vi "cdex - update quadcopter 3D model.vi"(5 "Y":sgl(slide) scale=-5.0..5.0, 7 "X":sgl(slide) scale=-5.0..5.0, 8 "Height":dbl(slide)=1.0 scale=0.0..4.0, 9 "Yaw":dbl(knob) scale=-6.28..6.28, 10 "Roll":dbl(knob) scale=-6.28..6.28, 11 "Pitch":dbl(knob) scale=-6.28..6.28) -> (3 "3D Picture Control":refnum<vi>(3d-picture))   [LabVIEW 2015]
uses:
  <vilib>/Analysis/1siggen.llb/Ramp Pattern by Samples.vi
  <vilib>/picture/3D Picture Control/NI_3D Picture Control.lvlib
  <vilib>/Analysis/NI_AALBase.lvlib
panel:
  # "Deploying Real-Time Math with NI LabVIEW"
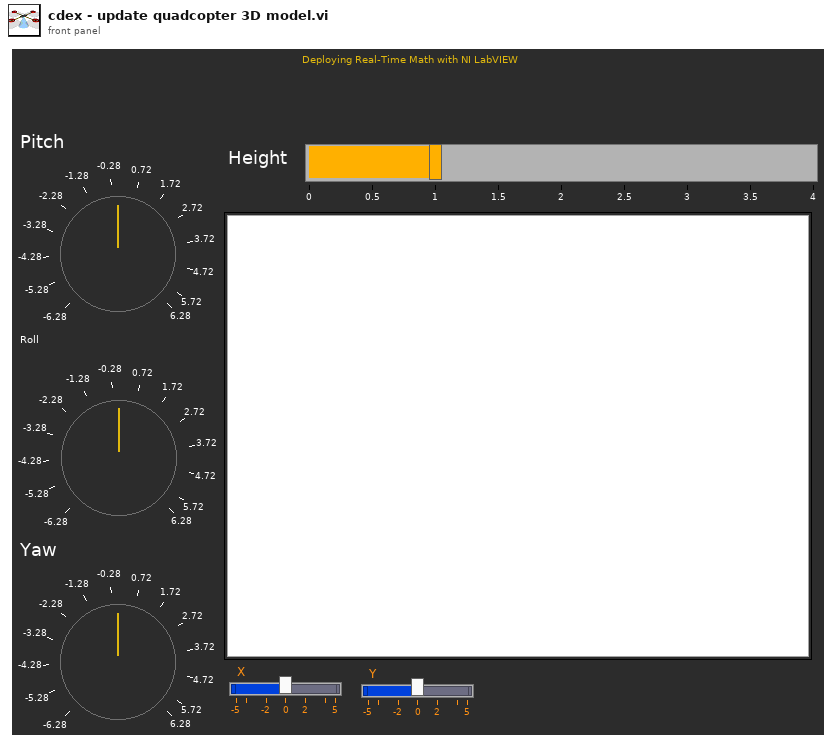
[diagram p1: front panel]
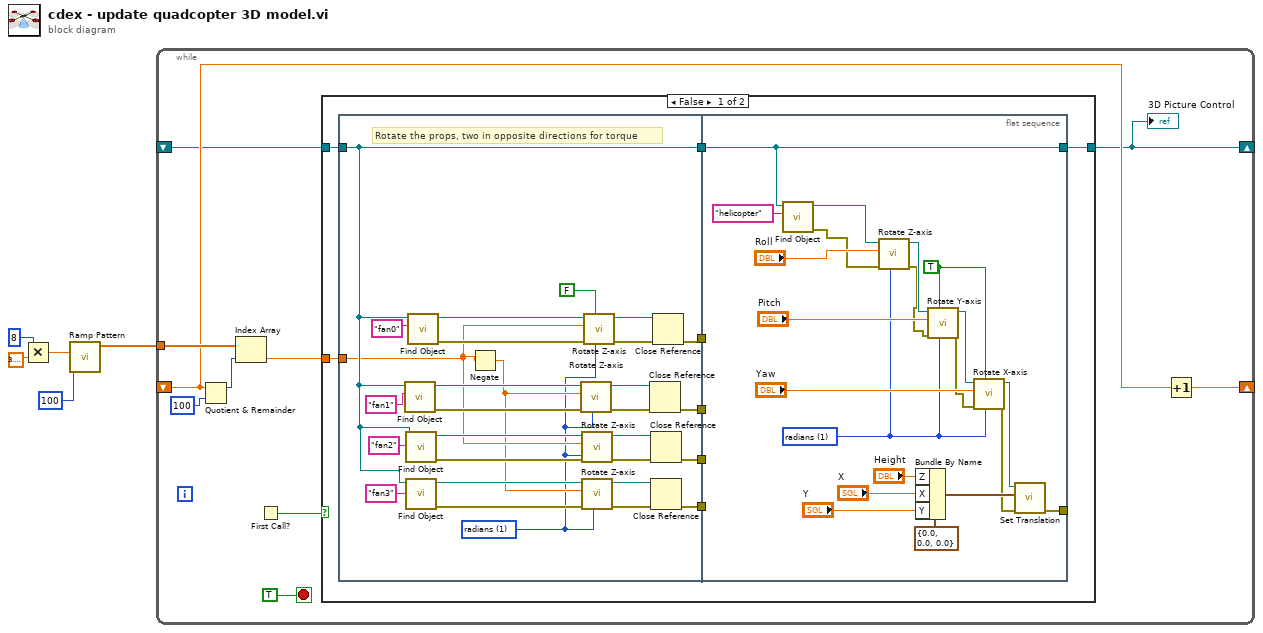
[diagram p0: block diagram]
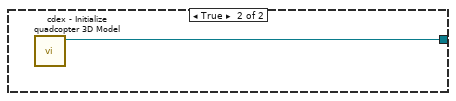
[diagram p2: hidden frame]
diagram:
  n1 = Multiply(x=8, y=3.141592653589793) -> (x*y=w3:dbl)
  n2 = call-poly <vilib>:"Ramp Pattern.vi"("end"=w3, "samples"=100) -> ("Ramp Pattern"=w1:dbl[])  [unwired: 8 in, 1 out]
  n3 = while {
    tunnel: w1 -> [w14]
    shift-right: [w11] -> _
    shift-left: _ -> [w10]
    shift-right: [w6] -> _
    shift-left: _ -> [w9]
    stop <- TRUE stop-if-true
    n4 = Quotient & Remainder(x=w10, y=100) -> (x-y*floor(x/y)=w13:i32)  [unwired: 1 out]
    n5 = Index Array(array=w14, index=w13) -> (element=w12:dbl)
    n6 = First Call?() -> (First Call?: T/F=w7:bool)
    n7 = case shown="False" w7 {
      tunnel: w9 -> [w22 _]
      tunnel: w12 -> [w21 _]
      tunnel: [w20 w74] -> w6
      frame False {
        n8 = flat-sequence {
          tunnel: w22 -> [w31]
          tunnel: [w31] -> w23
          tunnel: w21 -> [w30]
          tunnel: [w27] -> w19
          tunnel: [w26] -> w18
          tunnel: [w25] -> w17
          tunnel: [w24] -> w16
          tunnel: [w58] -> w20
          tunnel: w23 -> [w58]
          tunnel: w19 -> [_]
          tunnel: w18 -> [_]
          tunnel: w17 -> [_]
          tunnel: w16 -> [_]
          tunnel: [w53] -> _
          frame #0 {
            w28 = u16 1 items=["degree", "radians"] ("angle unit")
            # "Rotate the props, two in opposite directions for torque"
            n9 = call <vilib>:"Find Object.vi"("Object Name"="fan1", "Scene Refnum"=w31) -> ("error out"=w44:errorcluster, "Object Refnum"=w43:refnum<vi>)  [unwired: 8 in]
            n10 = call <vilib>:"Find Object.vi"("Object Name"="fan2", "Scene Refnum"=w31) -> ("error out"=w41:errorcluster, "Object Refnum"=w42:refnum<vi>)  [unwired: 8 in]
            n11 = call <vilib>:"Find Object.vi"("Object Name"="fan3", "Scene Refnum"=w31) -> ("error out"=w36:errorcluster, "Object Refnum"=w35:refnum<vi>)  [unwired: 8 in]
            n12 = call <vilib>:"Find Object.vi"("Object Name"="fan0", "Scene Refnum"=w31) -> ("error out"=w50:errorcluster, "Object Refnum"=w52:refnum<vi>)  [unwired: 8 in]
            n13 = Negate(x=w30) -> (-x=w29:dbl)
            n14 = call <vilib>:"Rotate Z-axis.vi"("angle unit"=w28, "error in (no error)"=w44, "angle"=w29, "Scene Object In"=w43) -> ("error out"=w46:errorcluster, "Scene Object Out"=w45:refnum<vi>)  [unwired: 6 in]
            n15 = call <vilib>:"Rotate Z-axis.vi"("angle unit"=w28, "error in (no error)"=w41, "angle"=w30, "Scene Object In"=w42) -> ("error out"=w39:errorcluster, "Scene Object Out"=w40:refnum<vi>)  [unwired: 6 in]
            n16 = call <vilib>:"Rotate Z-axis.vi"("angle unit"=w28, "error in (no error)"=w36, "angle"=w29, "Scene Object In"=w35) -> ("error out"=w38:errorcluster, "Scene Object Out"=w37:refnum<vi>)  [unwired: 6 in]
            n17 = call <vilib>:"Rotate Z-axis.vi"("angle unit"=w28, "Relative?"=FALSE, "error in (no error)"=w50, "angle"=w30, "Scene Object In"=w52) -> ("error out"=w47:errorcluster, "Scene Object Out"=w49:refnum<vi>)  [unwired: 5 in]
            n18 = Close Reference(reference=w45, error in (no error)=w46) -> (error out=w25:errorcluster)
            n19 = Close Reference(reference=w40, error in (no error)=w39) -> (error out=w26:errorcluster)
            n20 = Close Reference(reference=w37, error in (no error)=w38) -> (error out=w27:errorcluster)
            n21 = Close Reference(reference=w49, error in (no error)=w47) -> (error out=w24:errorcluster)
          }
          frame #1 {
            w59 = TRUE ("Relative?")
            w60 = u16 1 items=["degree", "radians"] ("angle unit")
            n22 = call <vilib>:"Find Object.vi"("Object Name"="helicopter", "Scene Refnum"=w58) -> ("error out"=w57:errorcluster, "Object Refnum"=w61:refnum<vi>)  [unwired: 8 in]
            n23 = call <vilib>:"Rotate Z-axis.vi"("angle unit"=w60, "error in (no error)"=w57, "angle"="Roll", "Scene Object In"=w61) -> ("error out"=w56:errorcluster, "Scene Object Out"=w73:refnum<vi>)  [unwired: 6 in]
            n24 = Bundle By Name(cluster=cluster{"X":sgl, "Y":sgl, "Z":sgl} {"X"=0.0, "Y"=0.0, "Z"=0.0} ("Axis"), "Z"="Height", "X"="X", "Y"="Y") -> (w70:cluster{"X":sgl, "Y":sgl, "Z":sgl})
            n25 = call <vilib>:"Rotate Y-axis.vi"("angle unit"=w60, "Relative?"=w59, "error in (no error)"=w56, "angle"="Pitch", "Scene Object In"=w73) -> ("error out"=w55:errorcluster, "Scene Object Out"=w72:refnum<vi>)  [unwired: 5 in]
            n26 = call <vilib>:"Rotate X-axis.vi"("angle unit"=w60, "Relative?"=w59, "error in (no error)"=w55, "angle"="Yaw", "Scene Object In"=w72) -> ("error out"=w54:errorcluster, "Scene Object Out"=w71:refnum<vi>)  [unwired: 5 in]
            n27 = call <vilib>:"Set Translation.vi"("error in (no error)"=w54, "Translation"=w70, "Scene Object"=w71) -> ("error out"=w53:errorcluster)  [unwired: 7 in, 1 out]
          }
        }
      }
      frame True {
        n28 = call "cdex - Initialize quadcopter 3D Model.vi"() -> ("Main Scene Object"=w74:refnum<vi>)  [unwired: 10 in, 1 out]
      }
    }
    "3D Picture Control" <- w6
    n29 = Increment(x=w10) -> (x+1=w11:dbl)
  }
